vi "Image Display Copy Image to Clipboard.vi"(8 "Error In":errorcluster, 9 "Image to Clipboard Options":T1={"Include Overlay (T)"=TRUE, "Image Only (T)"=TRUE}, 11 "Display Image Control Refnum":T2) -> (0 "Error Out":errorcluster)   [LabVIEW 2021, in "Image.lvlib"]
uses:
  Image Control Refnum.ctl
  Image Display to Clipboard Options.ctl
  Image.lvlib
panel:
  out "2D Picture":picture
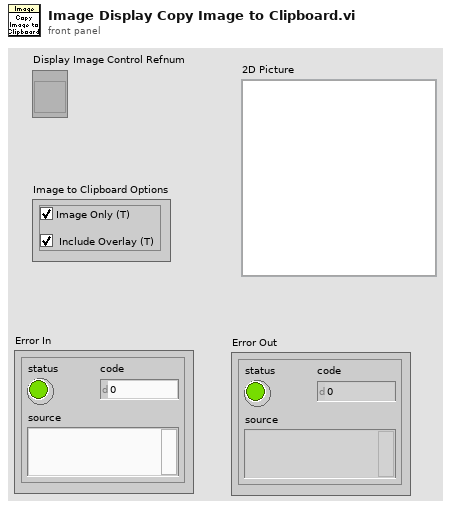
[diagram p1: front panel]
types:
  T1 = typedef "Image.lvlib/Image Display to Clipboard Options.ctl" = cluster{"Include Overlay (T)":bool, "Image Only (T)":bool}
  T2 = typedef "Image.lvlib/Image Control Refnum.ctl" = refnum<vi>
  T3 = typedef "imagedata.ctl" = cluster{"image type":i32, "image depth":i32, "image":u8[], "mask":u8[], "colors":u32[], "Rectangle":cluster{"left":i16, "top":i16, "right":i16, "bottom":i16}}
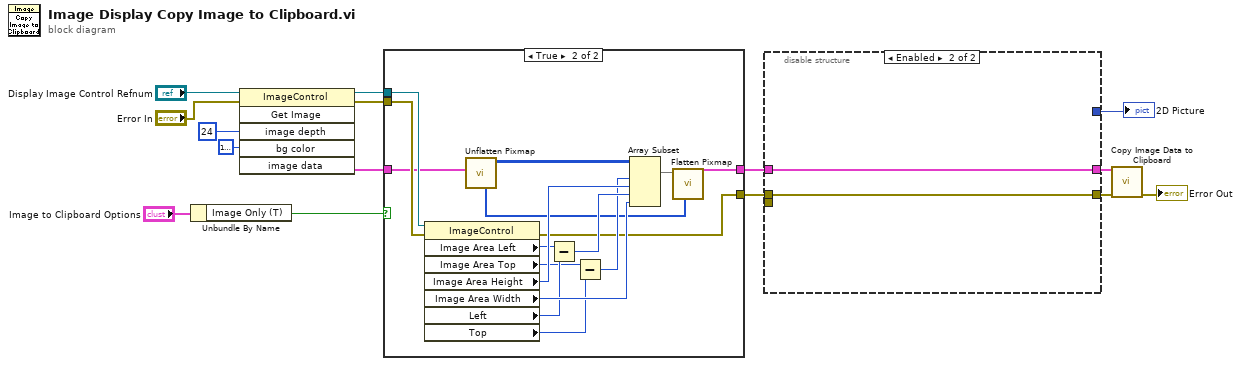
[diagram p0: block diagram]
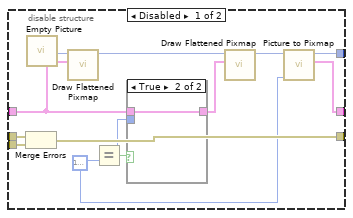
[diagram p2: hidden frame]
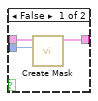
[diagram p3: hidden frame]
diagram:
  n1 = Unbundle By Name("Image to Clipboard Options") -> ("Image Only (T)"=w11:bool)
  n2 = invoke class="ImageControl" method="Get Image"(reference="Display Image Control Refnum", error in="Error In", "image depth"=24 ("Image Depth"), "bg color"=u32 16777226 ("Background Color")) -> (reference out=w8:T2, error out=w10:errorcluster, "image data"=w7:T3)  [unwired: 2 in, 3 out]
  n3 = case shown="True" w11 {
    tunnel: w10 -> [w17 w21]
    tunnel: [w17 w20] -> w9
    tunnel: [w16 w19] -> w4
    tunnel: w8 -> [_ w22]
    tunnel: w7 -> [w16 w18]
    frame False {
    }
    frame True {
      n4 = property class="ImageControl"(reference=w22, error in=w21) -> (error out=w20:errorcluster, "Image Area Left"=w24:i32, "Image Area Top"=w25:i32, "Image Area Height"=w32:u32, "Image Area Width"=w33:u32, "Left"=w28:i32, "Top"=w29:i32)  [unwired: 1 out]
      n5 = call <vilib>:"Unflatten Pixmap.vi"("image data"=w18) -> ("24-bit pixmap"=w23:u32[][], "colors"=w27:u32[])  [unwired: 4 in, 5 out]
      n6 = Subtract(x=w24, y=w28) -> (x-y=w31:i32)
      n7 = Subtract(x=w25, y=w29) -> (x-y=w30:i32)
      n8 = Array Subset(array=w23, index (row)=w30, length (row)=w32, index (col)=w31, length (col)=w33) -> (w26:u32[][])
      n9 = call <vilib>:"Flatten Pixmap.vi"("colors"=w27, "24-bit pixmap"=w26) -> ("image data"=w19:T3)  [unwired: 9 in]
    }
  }
  n10 = disable-structure shown="Enabled" {
    disable-tunnel: w9 -> [w46 w51]
    disable-tunnel: [w44 w51] -> w5
    disable-tunnel: _ -> [w43 _]
    disable-tunnel: w4 -> [w41 w52]
    disable-tunnel: [w36 w52] -> w3
    disable-tunnel: [w35 _] -> w2
    frame Disabled {
      w34 = u32 16777216 ("Mask Color (Black)")
      n11 = Merge Errors(w46, w43) -> (w44:errorcluster)
      n12 = call "Empty Picture"() -> ("empty picture"=w40:picture)
      n13 = call <vilib>:"Draw Flattened Pixmap.vi"("image data"=w41, "picture"=w40) -> ("new picture"=w39:picture)  [unwired: 7 in]
      n14 = Equal?(x=w42, y=w34) -> (x = y?=w45:bool)
      n15 = case shown="True" w45 {
        tunnel: w41 -> [w49 w50]
        tunnel: [w48 w50] -> w38
        tunnel: [w47 _] -> w42
        frame False {
          n16 = call <vilib>:"Create Mask.vi"("Mask Color (Black)"=w47, "image data"=w49) -> ("image data"=w48:T3)  [unwired: 9 in]
        }
        frame True {
        }
      }
      n17 = call <vilib>:"Draw Flattened Pixmap.vi"("image data"=w38, "picture"=w39) -> ("new picture"=w37:picture)  [unwired: 7 in]
      n18 = call <vilib>:"Picture to Pixmap.vi"("Background Color"=w34, "picture"=w37) -> ("image data"=w36:T3, "new picture"=w35:picture)  [unwired: 8 in]
    }
    frame Enabled {
    }
  }
  "2D Picture" <- w2
  n19 = call "Copy Image Data to Clipboard.vi"("error in (no error)"=w5, "image data"=w3) -> ("error out"=→"Error Out":errorcluster)  [unwired: 9 in]
